vi "User Event Generation.vi"() -> ()   [LabVIEW 2023]
doc: "Demonstrates User Events functions to implement a user interaction recorder. After moving the Slider value to different positions, you can press the Playback button to fire a series of User Events that will display the stored Slider values in the Movement Data graph.\n\nThis example shows a usage of the Simple State Machine project template."
uses:
  controls/User Event Record State.ctl
  controls/User Event Record Data.ctl
panel:
  out "Recording State":u16(ring) items=["Idle", "Recording", "Playback"]
  out "Movement Data":i16(graph)
  in  "Slider":i16(slide) scale=0.0..20.0
  in  "Stop":bool
  in  "Playback":bool
  # "Overview: Demonstrates the User Events functions to implement a user interaction recorder.\nInstructions:\n1. Run the VI.\n2. Drag the value of the Slider control around for a few seconds.\n3. Click the Playback button. The exact sequence of drags that you performed will be repeated on the Slider, and displayed in the Movement Data graph.\n4. Click Stop to stop the VI."
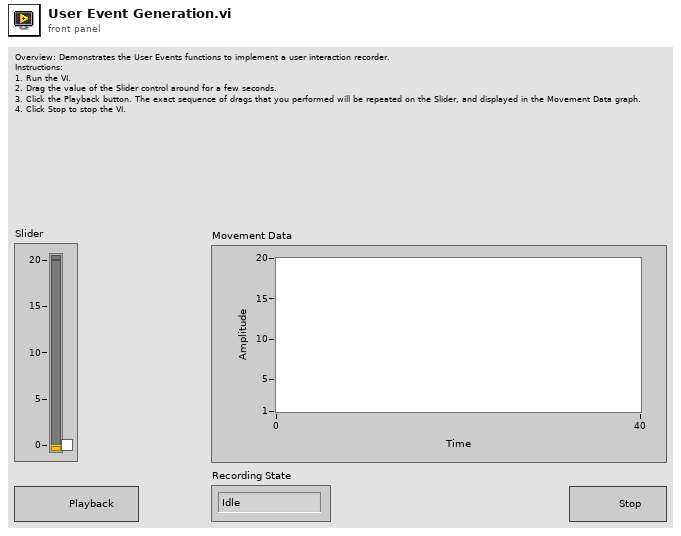
[diagram p1: front panel]
types:
  T1 = typedef "User Event Record Data.ctl" = cluster{"Position":i16, "Delay":u32}
  T2 = typedef "User Event Record State.ctl" = enum16{"Initialize", "Wait for Event", "Initiate Playback", "Exit"}
  T3 = enum8{"Enabled", "Disabled", "Disabled and Grayed Out"}
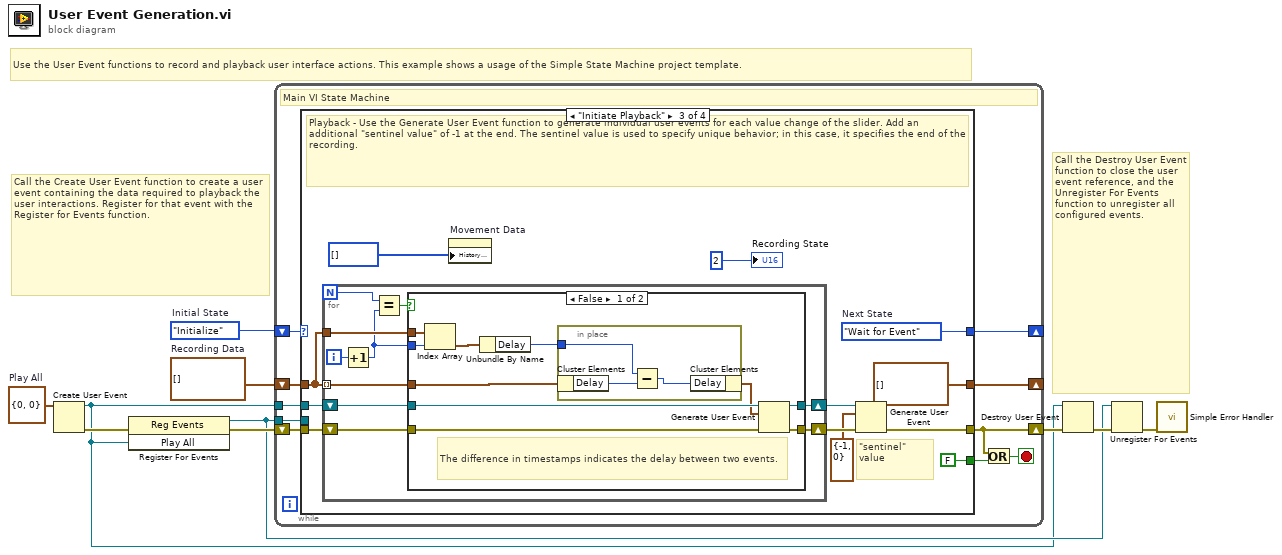
[diagram p0: block diagram]
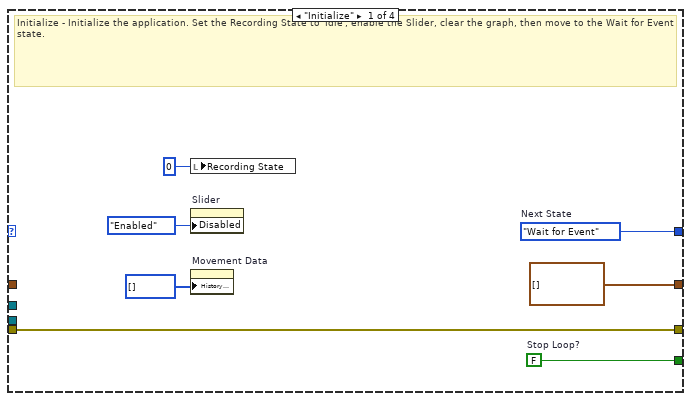
[diagram p2: hidden frame]
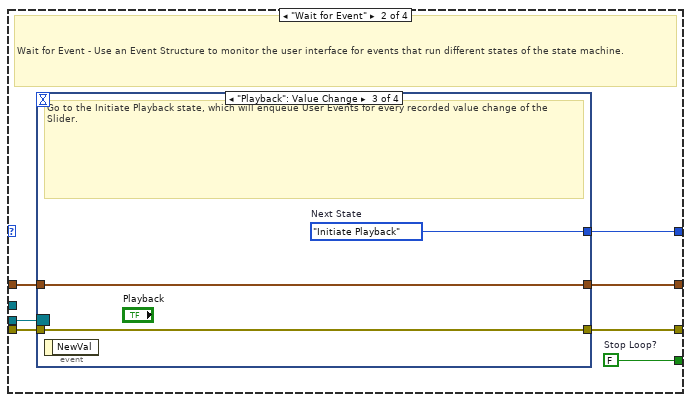
[diagram p3: hidden frame]
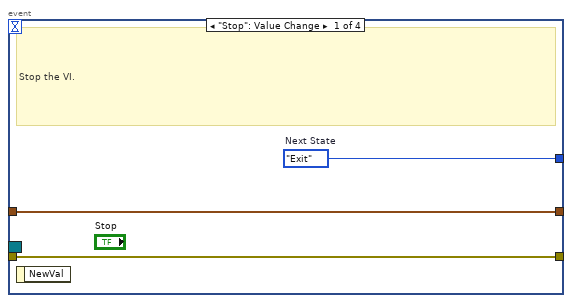
[diagram p4: hidden frame]
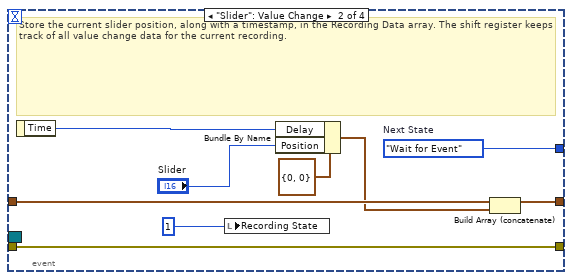
[diagram p5: hidden frame]
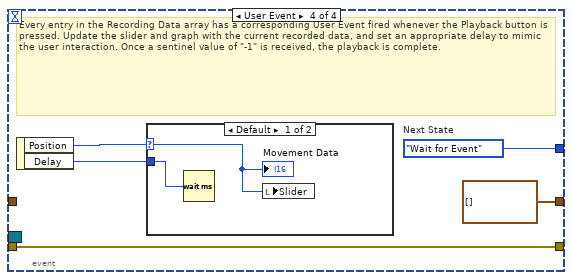
[diagram p6: hidden frame]
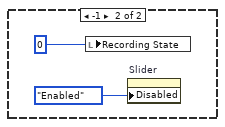
[diagram p7: hidden frame]
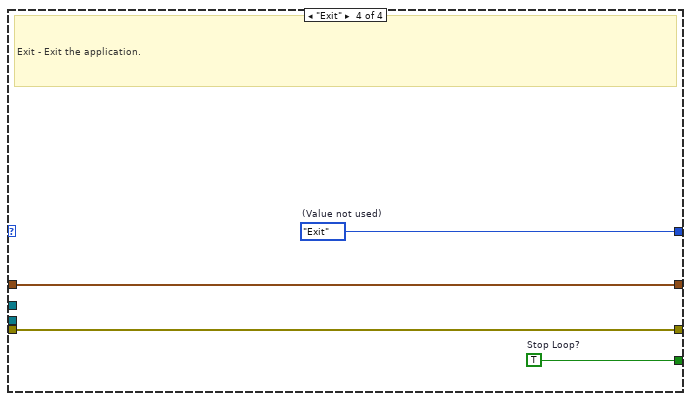
[diagram p9: hidden frame]
diagram:
  w8 = T1[] []  # Recording Data
  w5 = T1 {"Position"=0, "Delay"=0}  # Play All
  w10 = User_Event_Record_State."Initialize"  # Initial State
  # "Call the Create User Event function to create a user event containing the data required to playback the user interactions. Register for that event with the Register for Events function."
  # "Call the Destroy User Event function to close the user event reference, and the Unregister For Events function to unregister all configured events."
  # "Use the User Event functions to record and playback user interface actions. This example shows a usage of the Simple State Machine project template."
  n1 = Create User Event(user event datatype=w5) -> (user event=w1:refnum<user-event>, error out=w6:errorcluster)  [unwired: 1 in]
  n2 = register-events(error in=w6, w1) -> (reference out=w2:refnum<event-registration>, error out=w7:errorcluster)  [unwired: 1 in]
  n3 = while {
    shift-right: [w19] -> _
    shift-left: w10 -> [w20]
    shift-right: [w15] -> w9
    shift-left: w7 -> [w18]
    shift-right: [w13] -> _
    shift-left: w8 -> [w14]
    tunnel: w2 -> [w12]
    tunnel: w1 -> [w11]
    stop <- w16 stop-if-true
    # "Main VI State Machine"
    n4 = case shown="\"Initiate Playback\"" w20 {
      tunnel: [w25 w34 w69 w97] -> w19
      tunnel: [w27 w33 FALSE ("Stop Loop?") w99] -> w17
      tunnel: w18 -> [w26 w32 w67 w98]
      tunnel: [w26 w31 w63 w98] -> w15
      tunnel: w14 -> [_ w30 w61 w96]
      tunnel: [T1[] [] ("Recording Data") w29 T1[] [] ("Recording Data") w96] -> w13
      tunnel: w12 -> [_ w28 _ _]
      tunnel: w11 -> [_ _ w66 _]
      frame "Initialize" {
        w25 = User_Event_Record_State."Wait for Event"  # Next State
        w27 = FALSE  # Stop Loop?
        # "Initialize - Initialize the application. Set the Recording State to 'Idle', enable the Slider, clear the graph, then move to the Wait for Event state."
        n5 = local write "Recording State"(u16 0) -> ()
        n6 = property on="Slider" class="Slide (strict)"("Disabled"=T3."Enabled") -> ()  [unwired: 2 in, 2 out]
        n7 = property on="Movement Data" class="WFChart (strict)"("History Data"=i16[] []) -> ()  [unwired: 2 in, 2 out]
      }
      frame "Wait for Event" {
        w33 = FALSE  # Stop Loop?
        # "Wait for Event - Use an Event Structure to monitor the user interface for events that run different states of the state machine."
        n8 = event shown="[2] \"Playback\": Value Change" {
          selector: w28 -> [_ _ _ _]
          dyn-events: _ -> [_ _ _ _]
          timeout: _ -> [_ _ _ _]
          tunnel: [w36 w43 w48 w53] -> w34
          tunnel: w32 -> [w37 w46 w49 w54]
          tunnel: [w37 w46 w49 w54] -> w31
          tunnel: w30 -> [w35 w45 w47 _]
          tunnel: [w35 w44 w47 T1[] [] ("Recording Data")] -> w29
          event "Stop": Value Change {
            w36 = User_Event_Record_State."Exit"  # Next State
            # "Stop the VI."
            n9 = event-data() -> ()  [unwired: 1 in, 1 out]
          }
          event "Slider": Value Change {
            w43 = User_Event_Record_State."Wait for Event"  # Next State
            # "Store the current slider position, along with a timestamp, in the Recording Data array. The shift register keeps track of all value change data for the current recording."
            n10 = event-data() -> ("Time"=w41:u32)  [unwired: 1 in]
            n11 = local write "Recording State"(u16 1) -> ()
            n12 = Bundle By Name(cluster=T1 {"Position"=0, "Delay"=0} ("Record Data"), "Delay"=w41, "Position"="Slider") -> (w39:T1)
            n13 = Build Array (concatenate)(w45, w39) -> (w44:T1[])
          }
          event "Playback": Value Change {
            w48 = User_Event_Record_State."Initiate Playback"  # Next State
            # "Go to the Initiate Playback state, which will enqueue User Events for every recorded value change of the Slider."
            n14 = event-data() -> ()  [unwired: 1 in, 1 out]
          }
          event User Event {
            w53 = User_Event_Record_State."Wait for Event"  # Next State
            # "Every entry in the Recording Data array has a corresponding User Event fired whenever the Playback button is pressed. Update the slider and graph with the current recorded data, and set an appropriate delay to mimic the user interaction. Once a sentinel value of \"-1\" is received, the playback is complete."
            n15 = event-data() -> ("Position"=w51:i16, "Delay"=w50:u32)  [unwired: 1 in]
            n16 = case shown="Default" w51 {
              selector: w51 -> [w56 _]
              tunnel: w50 -> [w55 _]
              frame Default {
                n17 = Wait (ms)(milliseconds to wait=w55) -> ()  [unwired: 1 out]
                n18 = local write "Slider"(w56) -> ()
                "Movement Data" <- w56
              }
              frame -1 {
                n19 = local write "Recording State"(u16 0) -> ()
                n20 = property on="Slider" class="Slide (strict)"("Disabled"=T3."Enabled") -> ()  [unwired: 2 in, 2 out]
              }
            }
          }
        }
      }
      frame "Initiate Playback" {
        w69 = User_Event_Record_State."Wait for Event"  # Next State
        # "\"sentinel\" value"
        # "Playback - Use the Generate User Event function to generate individual user events for each value change of the slider. Add an additional \"sentinel value\" of -1 at the end. The sentinel value is used to specify unique behavior; in this case, it specifies the end of the recording."
        n21 = for {
          N -> [w73]
          tunnel: w61 -> [w79]
          shift-right: [w78] -> w65
          shift-left: w66 -> [w80]
          shift-right: [w76] -> w64
          shift-left: w67 -> [w77]
          tunnel: w61 -> [w74] mode=indexing
          i -> [w75]
          n22 = Increment(x=w75) -> (x+1=w72:i32)
          n23 = Equal?(x=w73, y=w72) -> (x = y?=w71:bool)
          n24 = case shown="False" w71 {
            tunnel: w80 -> [w90 w95]
            tunnel: w79 -> [w87 _]
            tunnel: [w86 w95] -> w78
            tunnel: w77 -> [w85 w94]
            tunnel: [w84 w94] -> w76
            tunnel: w74 -> [w83 _]
            tunnel: w72 -> [w81 _]
            frame False {
              # "The difference in timestamps indicates the delay between two events."
              n25 = Index Array(array=w87, index=w81) -> (element=w89:T1)
              n26 = Unbundle By Name(w89) -> ("Delay"=w88:u32)
              n27 = in-place {
                in-place-border: w88 -> [w93]
                n28 = in-place-cluster #1(w83) -> ("Delay"=w92:u32)
                n29 = Subtract(x=w93, y=w92) -> (x-y=w91:u32)
                n30 = in-place-cluster #1("Delay"=w91) -> (w82:T1)
              }
              n31 = Generate User Event(user event=w90, event data cluster=w82, error in=w85) -> (user event out=w86:refnum<user-event>, error out=w84:errorcluster)  [unwired: 1 in]
            }
            frame True {
              # "User events are fired for the time between each movement. Thus, this loop will run one iteration more than necessary. Ignore the last iteration."
            }
          }
        }
        n32 = property on="Movement Data" class="WFChart (strict)"("History Data"=i16[] []) -> ()  [unwired: 2 in, 2 out]
        n33 = Generate User Event(user event=w65, event data cluster=T1 {"Position"=-1, "Delay"=0} ("Record Data"), error in=w64) -> (error out=w63:errorcluster)  [unwired: 1 in, 1 out]
        "Recording State" <- u16 2
      }
      frame "Exit" {
        w97 = User_Event_Record_State."Exit"  # (Value not used)
        w99 = TRUE  # Stop Loop?
        # "Exit - Exit the application."
      }
    }
    n34 = Or(x=w15, y=w17) -> (x .or. y?=w16:bool)
  }
  n35 = Destroy User Event(user event=w1, error in=w9) -> (error out=w4:errorcluster)
  n36 = Unregister For Events(event registration refnum=w2, error in=w4) -> (error out=w3:errorcluster)
  n37 = call <vilib>:"Simple Error Handler.vi"("error in (no error)"=w3) -> ()  [unwired: 4 in, 5 out]
